vi "Test Draw Text ARGB.vi"(8 "error in (no error)":errorcluster, 11 "Test Case In":refnum<class "Image.lvclass">) -> (0 "error out":errorcluster, 3 "Test Case Out":refnum<class "Image.lvclass">)   [LabVIEW 2020, in "test.lvlib" / "Image.lvclass"]
uses:
  Image.lvclass
  C:/Program Files (x86)/National Instruments/LabVIEW 2020/vi.lib/Astemes/LUnit/Test Case.lvclass
  image/ARGB Colour.ctl
  image/Text Drawing Settings.ctl
  image/Font Face.ctl
  common/Image Point (Integer).ctl
  common/Image Size (Integer).ctl
  <vilib>/Astemes/LUnit/Test Case.lvclass/Test Case.ctl
  image/New Image (ARGB).vi
  4993e8ee-a06a-463a-9684-69129f64d5ce.vi
  image/New Image (ARGB).vi/3321fa97-f432-4e1e-8db9-a0df79aed21b.vi
  image/ARGB Colour to U32 Pixel Value.vi
  image/Draw Text (ARGB).vi/0015c4fc-6a12-4f82-815b-6c2f827f408b.vi
  image/Draw Image to Picture (ARGB).vi/8cd07b1b-062e-4fe4-9e87-2eb3dc89fe0e.vi
  <vilib>/Astemes/LUnit/Append Pass Result.vi
  <vilib>/Astemes/LUnit/Append Fail Result.vi
  <vilib>/Astemes/LUnit/Describe Comparison.vi
  4993e8ee-a06a-463a-9684-69129f64d5ce.vi/9c5d11cd-9439-4240-a1ee-d9baace9c924.vi
  <vilib>/Astemes/LUnit/Run In UI.vi
  <vilib>/Utility/error.llb/Clear Errors.vi
  common/Module Path.vi
  <vilib>/Utility/error.llb/Error Cluster From Error Code.vi
  <vilib>/Astemes/LUnit/Describe Variant.vi
  image/image.lvlib
  common/common.lvlib
panel:
  out "Picture":picture
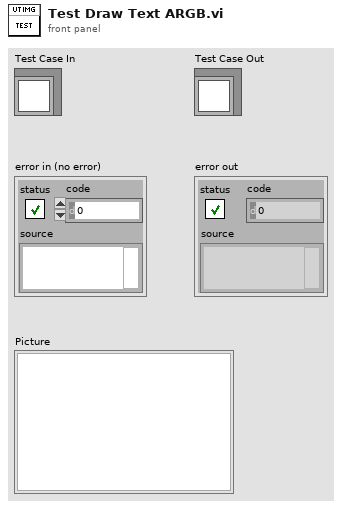
[diagram p1: front panel]
types:
  T1 = typedef "common.lvlib/Image Size (Integer).ctl" = cluster{"Width":u16, "Height":u16}
  T2 = typedef "common.lvlib/Image Point (Integer).ctl" = cluster{"x":i32, "y":i32}
  T3 = typedef "image.lvlib/Text Drawing Settings.ctl" = cluster{"OpenCV Font Face":T4, "Font Scale":dbl}
  T4 = typedef "image.lvlib/Font Face.ctl" = enum8{"FONT_HERSHEY_SIMPLEX", "FONT_HERSHEY_PLAIN", "FONT_HERSHEY_DUPLEX", "FONT_HERSHEY_COMPLEX", "FONT_HERSHEY_TRIPLEX", "FONT_HERSHEY_COMPLEX_SMALL", "FONT_HERSHEY_SCRIPT_SIMPLEX", "FONT_HERSHEY_SCRIPT_COMPLEX", "FONT_ITALIC"}
  T5 = typedef "image.lvlib/ARGB Colour.ctl" = cluster{"Alpha":u8, "RGB":u32}
  T6 = typedef "image.lvlib/ARGB Image.ctl" = refnum<data-value>
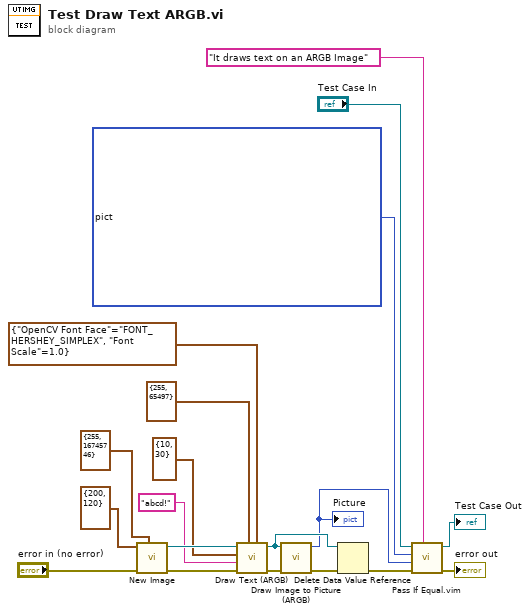
[diagram p0: block diagram]
diagram:
  n1 = call-poly "New Image.vi"("Colour (Default: Black)"=T5 {"Alpha"=255, "RGB"=16745746}, "error in (no error)"="error in (no error)", "Preallocated Image Size (Default: 0,0)"=T1 {"Width"=200, "Height"=120}) -> ("error out"=w12:errorcluster, "New ARGB Image"=w13:T6)  [unwired: 7 in]
  n2 = call "Draw Text (ARGB).vi"("Text Drawing Settings (Default: Simplex)"=T3 {"OpenCV Font Face"=enum."FONT_HERSHEY_SIMPLEX", "Font Scale"=1.0} ("Text Drawing Settings (Default: Simplex, Top-Left)"), "ARGB Colour"=T5 {"Alpha"=255, "RGB"=65497}, "error in (no error)"=w12, "Text"="abcd!", "Origin"=T2 {"x"=10, "y"=30}, "ARGB Image"=w13) -> ("error out"=w10:errorcluster, "ARGB Image (Duplicate)"=w11:T6)  [unwired: 4 in]
  n3 = call "Draw Image to Picture (ARGB).vi"("error in (no error)"=w10, "ARGB Image Source"=w11) -> ("error out"=w9:errorcluster, "Picture"=w7:picture)  [unwired: 8 in]
  "Picture" <- w7
  n4 = Delete Data Value Reference(data value reference=w11, error in=w9) -> (error out=w15:errorcluster)  [unwired: 1 out]
  n5 = call "Pass If Equal.vim"("Description"="It draws text on an ARGB Image", "error in (no error)"=w15, "Actual"=w7, "Expected"=picture bytes[72030] ("Picture"), "LUnit Test Case In"="Test Case In") -> ("error out"=→"error out":errorcluster, "LUnit Test Case Out"=→"Test Case Out":refnum<class "Image.lvclass">)  [unwired: 5 in]
